vi "Boolean_To_String.vi"(11 "16 bIT":bool[](array[boolean])) -> (3 "concatenated string 2":string)   [LabVIEW 2023]
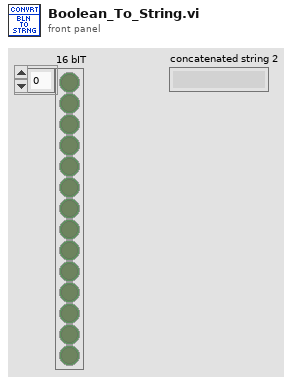
[diagram p1: front panel]
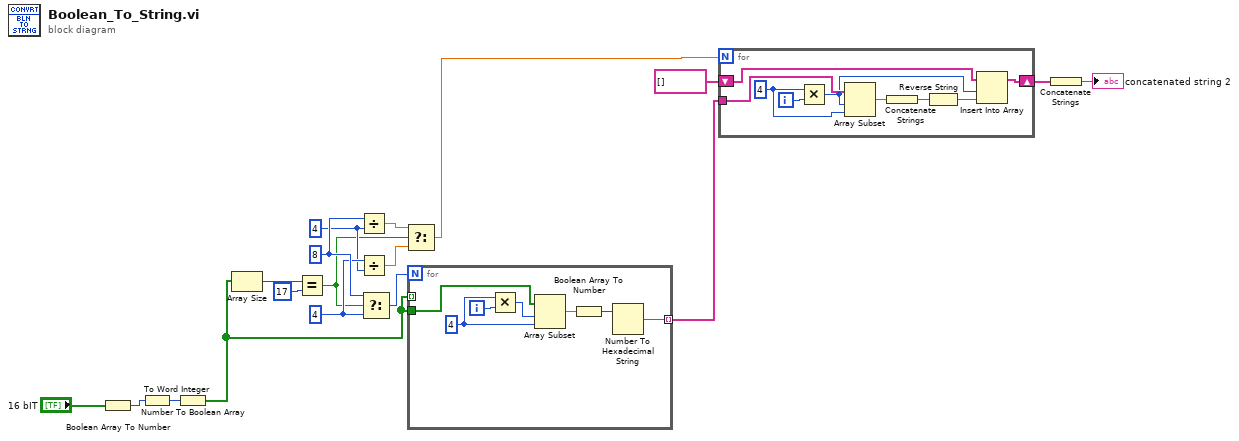
[diagram p0: block diagram]
diagram:
  w10 = 4 ("y")
  w11 = 4 ("y")
  w12 = 8 ("y")
  n1 = Boolean Array To Number(Boolean array="16 bIT") -> (number=w4:u32)
  n2 = To Word Integer(number=w4) -> (16bit integer=w3:i16)
  n3 = Number To Boolean Array(number=w3) -> (Boolean array=w1:bool[])
  n4 = Array Size(array=w1) -> (size(s)=w15:i32)
  n5 = Equal?(x=w15, y=17) -> (x = y?=w9:bool)
  n6 = Divide(x=w12, y=w10) -> (x/y=w8:dbl)
  n7 = Divide(x=w11, y=w10) -> (x/y=w7:dbl)
  n8 = Select(t=w12, s=w9, f=w11) -> (s? t:f=w13:i32)
  n9 = Select(t=w8, s=w9, f=w7) -> (s? t:f=w6:dbl)
  n10 = for {
    N: w13 -> [_]
    tunnel: w1 -> [w19]
    tunnel: [w20] -> w5 mode=indexing
    tunnel: w1 -> [_] mode=indexing
    i -> [w25]
    w24 = 4 ("length")
    n11 = Multiply(x=w24, y=w25) -> (x*y=w23:i32)
    n12 = Array Subset(array=w19, index=w23, length=w24) -> (w22:bool[])
    n13 = Boolean Array To Number(Boolean array=w22) -> (number=w21:u32)
    n14 = Number To Hexadecimal String(2:w21) -> (0:w20:string)  [unwired: 1 in]
  }
  n15 = for {
    N: w6 -> [_]
    tunnel: w5 -> [w34]
    shift-right: [w30] -> w17
    shift-left: string[] [] ("array") -> [w31]
    i -> [w32]
    w33 = 4 ("length")
    n16 = Multiply(x=w33, y=w32) -> (x*y=w29:i32)
    n17 = Array Subset(array=w34, index=w29, length=w33) -> (w28:string[])
    n18 = Concatenate Strings(w28) -> (w27:string)
    n19 = Reverse String(1:w27) -> (0:w26:string)
    n20 = Insert Into Array(array=w31, index=w29, new element=w26) -> (w30:string[])
  }
  n21 = Concatenate Strings(w17) -> (→"concatenated string 2":string)
